vi "Read Client type.vi"(8 "error in (no error)":errorcluster, 11 "Client in":refnum<class "PD-Client.lvclass">) -> (0 "error out":errorcluster, 2 "Client type":string, 3 "Client out":refnum<class "PD-Client.lvclass">)   [LabVIEW 2013, in "PowderDeposition.lvlib" / "PD-Client.lvclass"]
uses:
  PD-Client.lvclass
  PD-Client.lvclass/PD-Client.ctl
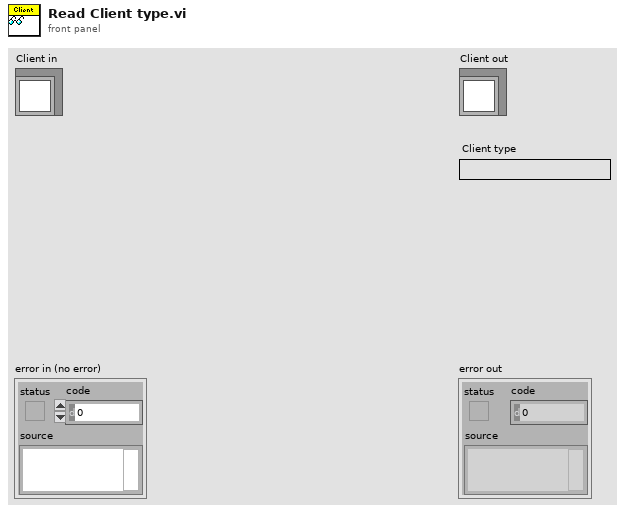
[diagram p1: front panel]
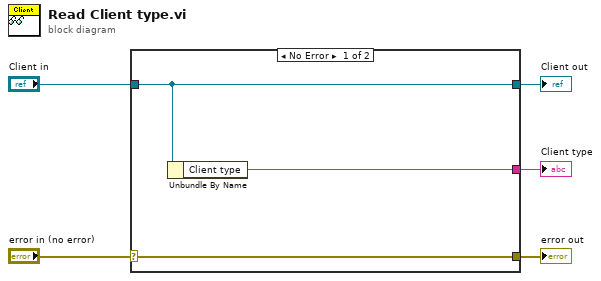
[diagram p0: block diagram]
diagram:
  n1 = case shown="No Error" "error in (no error)" {
    selector: "error in (no error)" -> [w8 w9]
    tunnel: [w8 w9] -> w4
    tunnel: [w7 w10] -> w2
    tunnel: "Client in" -> [w7 w10]
    tunnel: [w6 _] -> w1
    frame No Error {
      n2 = Unbundle By Name(w7) -> ("Client type"=w6:string)
    }
    frame Error {
    }
  }
  "error out" <- w4
  "Client out" <- w2
  "Client type" <- w1
